vi "Insert On.vi"(8 "error in (no error)":errorcluster, 9 "Item Tag":string, 10 "Tree Refnum":refnum<vi>, 11 "Tree Click Interpreter in":refnum<class "Tree Click Interpreter.lvclass">) -> (0 "error out":errorcluster, 1 "Insertion Index":i32, 2 "Parent ID":string, 3 "Tree Click Interpreter out":refnum<class "Tree Click Interpreter.lvclass">)   [LabVIEW 2017, in "Tree Click Interpreter.lvclass"]
uses:
  <vilib>/gpm_packages/@cs/Test-executive-builder/Source/Test Executive Builder View/Tree Click Interpreter/Tree Click Interpreter.lvclass
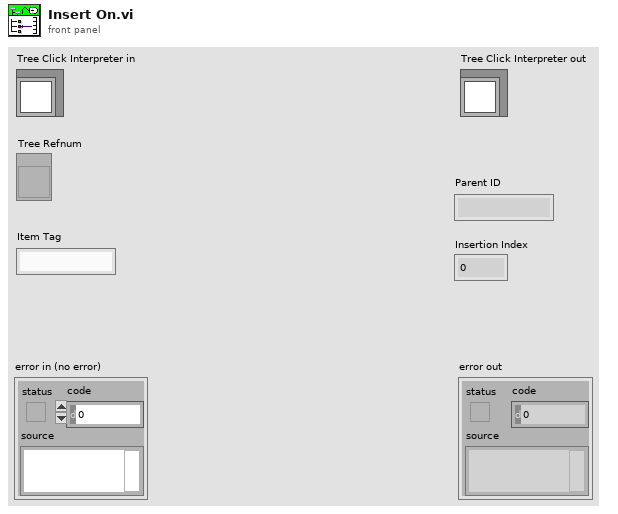
[diagram p1: front panel]
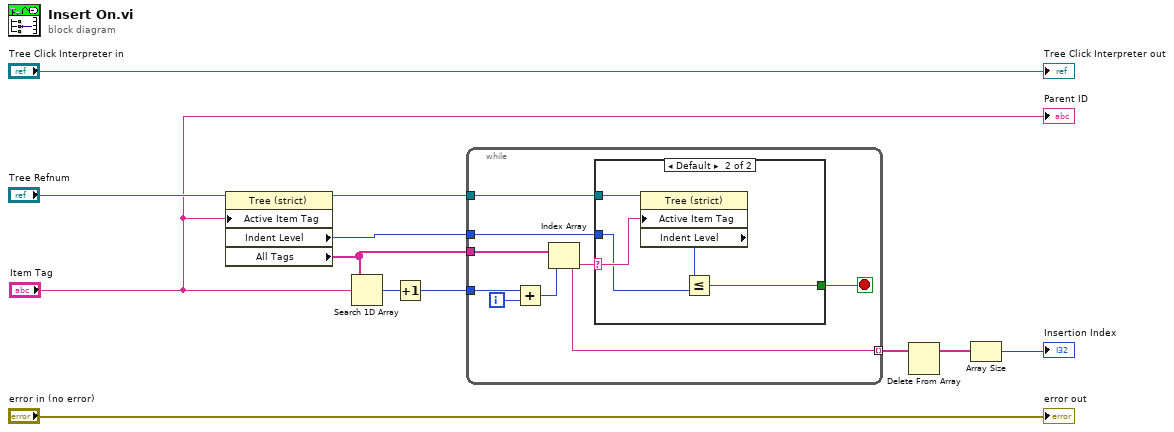
[diagram p0: block diagram]
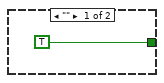
[diagram p2: hidden frame]
diagram:
  n1 = property class="Tree (strict)"(reference="Tree Refnum", "Active Item Tag"="Item Tag") -> (reference out=w4:refnum<vi>, "Indent Level"=w6:i32, "All Tags"=w5:string[])  [unwired: 1 in, 1 out]
  n2 = Search 1D Array(1D array=w5, element="Item Tag") -> (index of element=w8:i32)  [unwired: 1 in]
  n3 = Increment(x=w8) -> (x+1=w7:i32)
  n4 = while {
    tunnel: w7 -> [w20]
    tunnel: w6 -> [w15]
    tunnel: w5 -> [w18]
    tunnel: w4 -> [w14]
    tunnel: [w13] -> w3 mode=indexing
    i -> [w19]
    stop <- w16 stop-if-true
    n5 = Add(x=w20, y=w19) -> (x+y=w17:i32)
    n6 = Index Array(array=w18, index=w17) -> (element=w13:string)
    n7 = case shown="Default" w13 {
      selector: w13 -> [_ w25]
      tunnel: [TRUE w23] -> w16
      tunnel: w15 -> [_ w22]
      tunnel: w14 -> [_ w26]
      frame "" {
      }
      frame Default {
        n8 = property class="Tree (strict)"(reference=w26, "Active Item Tag"=w25) -> ("Indent Level"=w24:i32)  [unwired: 1 in, 2 out]
        n9 = Less Or Equal?(x=w24, y=w22) -> (x <= y?=w23:bool)
      }
    }
  }
  n10 = Delete From Array(array=w3) -> (array with subset deleted=w2:string[])  [unwired: 2 in, 1 out]
  n11 = Array Size(array=w2) -> (size(s)=→"Insertion Index":i32)
  "error out" <- "error in (no error)"
  "Tree Click Interpreter out" <- "Tree Click Interpreter in"
  "Parent ID" <- "Item Tag"
